vi "add pre post build to project.vi"(8 "error in (no error)":errorcluster, 9 "post build action vi":path, 10 "pre build action vi":path, 11 "Project in":refnum<vi>) -> (0 "error out":errorcluster, 2 "pre and post build refs":refnum<vi>[](array[refnum]), 3 "Project out":refnum<vi>)   [LabVIEW 2024]
doc: "If the path is valid, adds the pre and post build spec action vis to the open lv project"
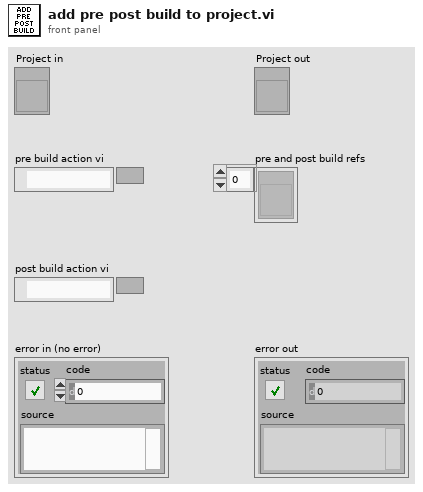
[diagram p1: front panel]
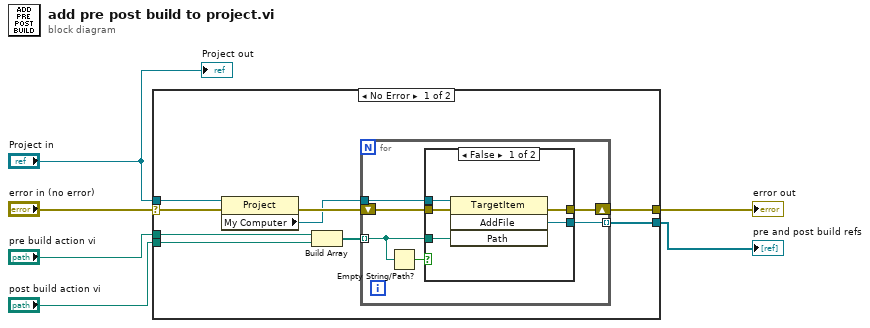
[diagram p0: block diagram]
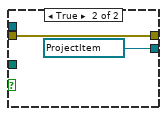
[diagram p2: hidden frame]
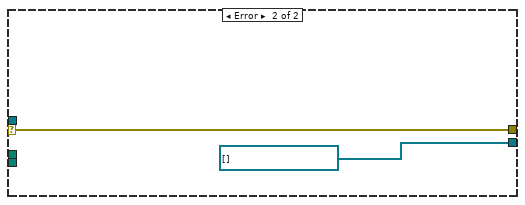
[diagram p3: hidden frame]
diagram:
  n1 = case shown="No Error" "error in (no error)" {
    selector: "error in (no error)" -> [w14 w30]
    tunnel: [w15 w30] -> w6
    tunnel: [w13 refnum<vi>[] []] -> w4
    tunnel: "post build action vi" -> [w12 _]
    tunnel: "Project in" -> [w10 _]
    tunnel: "pre build action vi" -> [w9 _]
    frame No Error {
      n2 = property class="Project"(reference=w10, error in=w14) -> (error out=w8:errorcluster, "My Computer"=w7:refnum<vi>)  [unwired: 1 out]
      n3 = Build Array(w9, w12) -> (w11:path[])
      n4 = for {
        tunnel: w7 -> [w21]
        tunnel: w11 -> [w18] mode=indexing
        tunnel: [w19] -> w13 mode=indexing
        shift-right: [w16] -> w15
        shift-left: w8 -> [w20]
        n5 = Empty String/Path?(string/path=w18) -> (empty?=w17:bool)
        n6 = case shown="False" w17 {
          tunnel: w21 -> [w26 _]
          tunnel: w20 -> [w25 w27]
          tunnel: w18 -> [w24 _]
          tunnel: [w23 refnum<vi> refnum ("AddFile")] -> w19
          tunnel: [w22 w27] -> w16
          frame False {
            n7 = invoke class="TargetItem" method="AddFile"(reference=w26, error in=w25, "Path"=w24) -> (error out=w22:errorcluster, "AddFile"=w23:refnum<vi>)  [unwired: 1 in, 2 out]
          }
          frame True {
          }
        }
      }
    }
    frame Error {
    }
  }
  "error out" <- w6
  "pre and post build refs" <- w4
  "Project out" <- "Project in"
